vi "Rotational button press.vi"(10 "Anticlockwise":bool, 11 "Clockwise":bool) -> (3 "rotDirection":dbl)   [LabVIEW 2017]
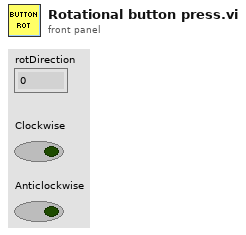
[diagram p1: front panel]
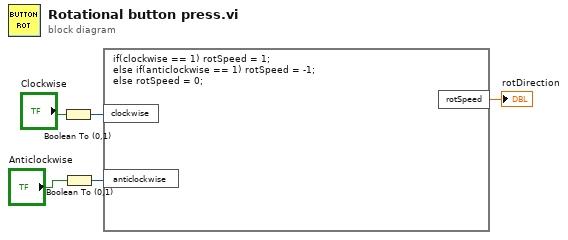
[diagram p0: block diagram]
diagram:
  n1 = Boolean To (0,1)(Boolean="Clockwise") -> (0, 1=w3:i16)
  n2 = Boolean To (0,1)(Boolean="Anticlockwise") -> (0, 1=w2:i16)
  n3 = formula code="if(clockwise == 1) rotSpeed = 1;\nelse if(anticlockwise == 1) rotSpeed = -1;\nelse rotSpeed = 0;"("anticlockwise"=w2, "clockwise"=w3) -> ("rotSpeed"=→"rotDirection":dbl)
